vi "ttm_aecontrolnew_poller.vi"() -> ()   [LabVIEW 2011]
panel:
  out "On AE speed":bool=TRUE
  out "Axis Information Out":T1(array[cluster])
  out "Axis Selector Out":i32[](listbox)
  out "Channels Out":u16[](array[ring]) items=["Channel 1", "Channel 2", "Channel 3", "Channel 4"]
  out "Error Out":errorcluster
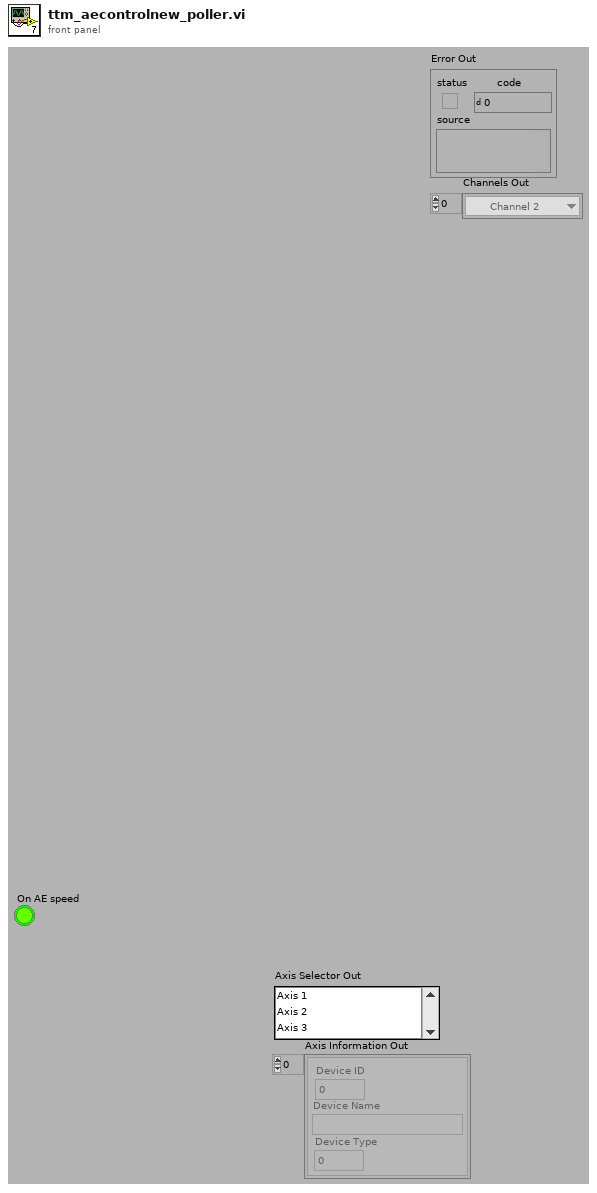
[diagram p1: front panel]
types:
  T1 = cluster{"Device ID":i32, "Device Name":string, "Device Type":i32}[]
  T2 = cluster{"Name":string, "Type":i32, "SI Full Scale":dbl, "Full Scale":dbl, "Units String":string, "Display Format":string, "Gauge Length":dbl}[][]
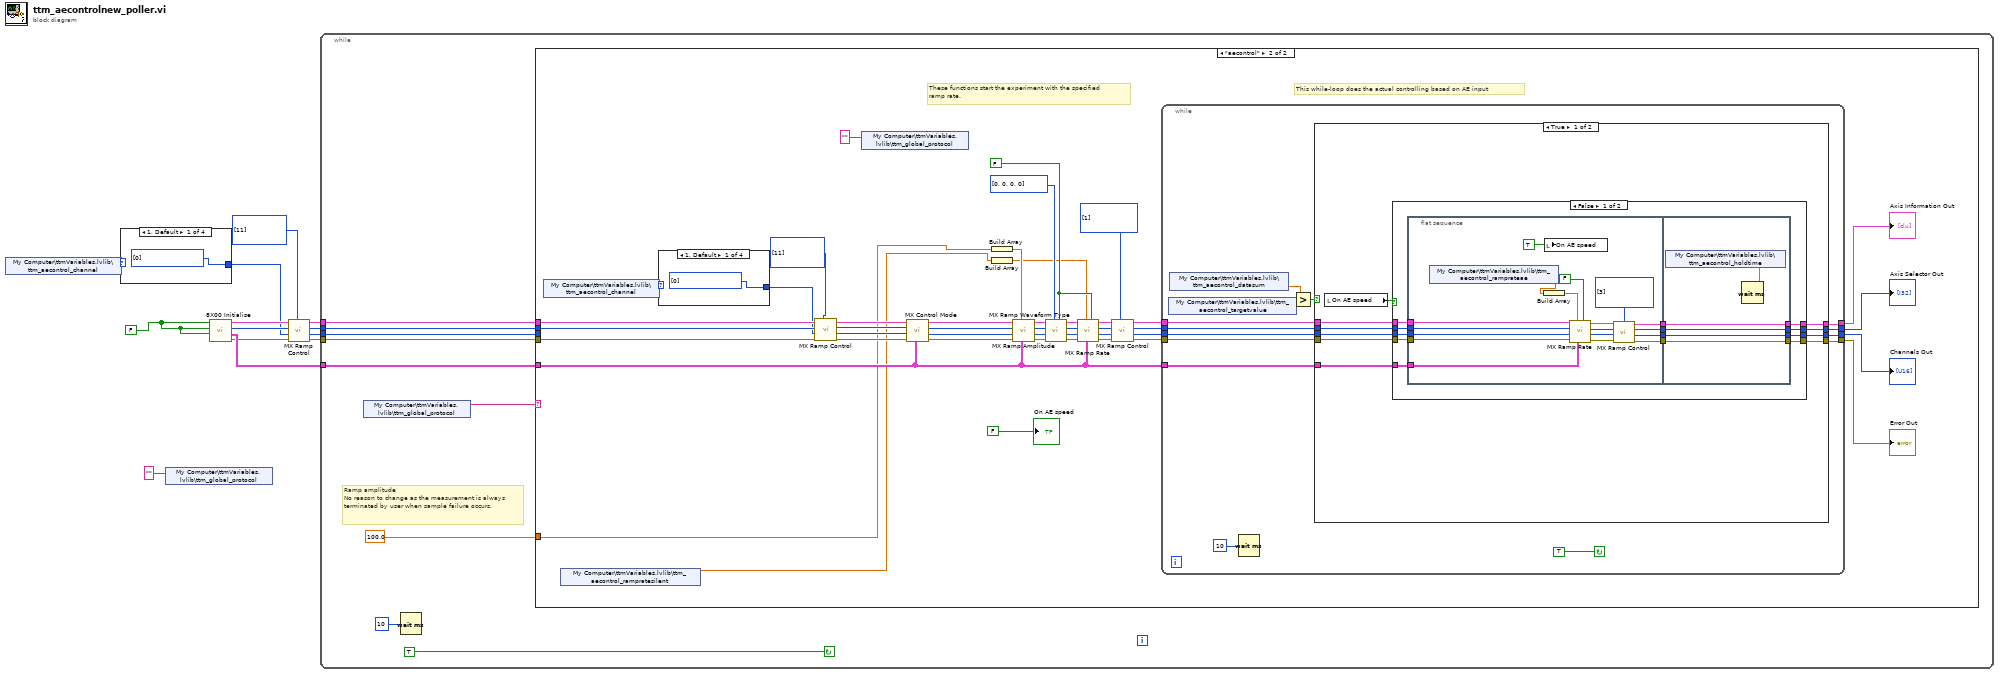
[diagram p0: block diagram]
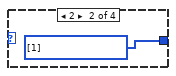
[diagram p2: hidden frame]
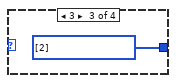
[diagram p3: hidden frame]
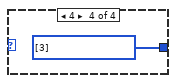
[diagram p4: hidden frame]
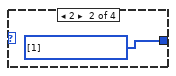
[diagram p6: hidden frame]
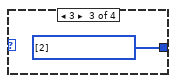
[diagram p7: hidden frame]
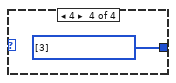
[diagram p8: hidden frame]
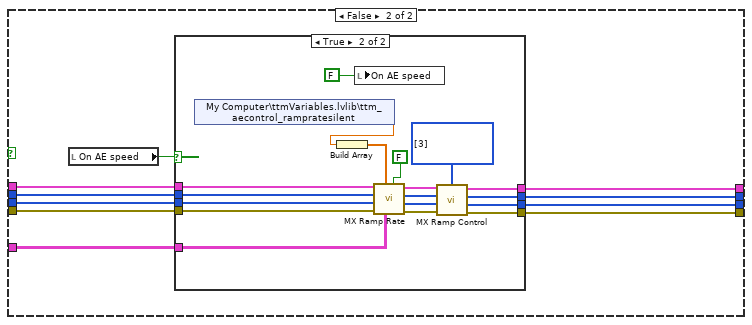
[diagram p10: hidden frame]
diagram:
  w7 = u16[] [11] items=["Stop", "Start or continue", "Hold", "Continue", "Return ramp to set level at fixed rate", "Reserved", "Reserved", "Start Random without demand hold", "Start Random with demand hold", "Prepare Random Start without demand hold", "Prepare Random Start with demand hold", "Unslave", "Reserved", "Reserved", "Start Sample Data Playback or Resume", "Prepare for Start of Sample Data", "Reserved", "Reserved", "Resume Playback", "Start an electromechanical frame return"] ("Ramp Control")
  w12 = FALSE ("Reset?")
  n1 = shared-variable "My Computer\\ttmVariables.lvlib\\ttm_aecontrol_channel"() -> (w9:i32)  [unwired: 1 in, 1 out]
  n2 = case shown="1, Default" w9 {
    tunnel: [w14 w15 w16 w17] -> w8
    frame 1, Default {
      w14 = u16[] [0] items=["Channel 1", "Channel 2", "Channel 3", "Channel 4"] ("Choose channel to apply\nthe setpoint")
    }
    frame 2 {
      w15 = u16[] [1] items=["Channel 1", "Channel 2", "Channel 3", "Channel 4"] ("Choose channel to apply\nthe setpoint")
    }
    frame 3 {
      w16 = u16[] [2] items=["Channel 1", "Channel 2", "Channel 3", "Channel 4"] ("Choose channel to apply\nthe setpoint")
    }
    frame 4 {
      w17 = u16[] [3] items=["Channel 1", "Channel 2", "Channel 3", "Channel 4"] ("Choose channel to apply\nthe setpoint")
    }
  }
  n3 = shared-variable "My Computer\\ttmVariables.lvlib\\ttm_global_protocol"("" ("protocol")) -> ()  [unwired: 1 in, 1 out]
  n4 = call "8X00 Initialise.vi"("Reset?"=w12, "Create DVM? (T)"=w12, "Create Console? (T)"=w12) -> ("error out"=w6:errorcluster, "Channel Data"=w13:T2, "Axis Selector"=w10:i32[], "Axis Information"=w11:T1)  [unwired: 1 in]
  n5 = call "MX Ramp Control.vi"("Ramp Control"=w7, "error in (no error)"=w6, "Channels In"=w8, "Axis Selector In"=w10, "Axis Information In"=w11) -> ("error out"=w2:errorcluster, "Channels Out"=w3:u16[], "Axis Selector Out"=w4:i32[], "Axis Information Out"=w5:T1)  [unwired: 2 in]
  n6 = while {
    tunnel: w13 -> [w25]
    tunnel: w5 -> [w22]
    tunnel: w4 -> [w21]
    tunnel: w3 -> [w20]
    tunnel: w2 -> [w19]
    stop <- TRUE continue-if-true
    # "Ramp amplitude\nNo reason to change as the measurement is always terminated by user when sample failure occurs."
    n7 = shared-variable "My Computer\\ttmVariables.lvlib\\ttm_global_protocol"() -> (w18:string)  [unwired: 1 in, 1 out]
    n8 = Wait (ms)(milliseconds to wait=u32 10) -> ()  [unwired: 1 out]
    n9 = case shown="\"aecontrol\"" w18 {
      tunnel: w25 -> [_ w41]
      tunnel: 100.0 ("rampAmplitude") -> [_ w28]
      tunnel: w22 -> [_ w37]
      tunnel: w21 -> [_ w36]
      tunnel: w20 -> [_ _]
      tunnel: w19 -> [_ w35]
      frame "False", Default {
      }
      frame "aecontrol" {
        w29 = u16[] [11] items=["Stop", "Start or continue", "Hold", "Continue", "Return ramp to set level at fixed rate", "Reserved", "Reserved", "Start Random without demand hold", "Start Random with demand hold", "Prepare Random Start without demand hold", "Prepare Random Start with demand hold", "Unslave", "Reserved", "Reserved", "Start Sample Data Playback or Resume", "Prepare for Start of Sample Data", "Reserved", "Reserved", "Resume Playback", "Start an electromechanical frame return"] ("Ramp Control")
        w50 = u16[] [1] items=["Stop", "Start or continue", "Hold", "Continue", "Return ramp to set level at fixed rate", "Reserved", "Reserved", "Start Random without demand hold", "Start Random with demand hold", "Prepare Random Start without demand hold", "Prepare Random Start with demand hold", "Unslave", "Reserved", "Reserved", "Start Sample Data Playback or Resume", "Prepare for Start of Sample Data", "Reserved", "Reserved", "Resume Playback", "Start an electromechanical frame return"] ("Ramp Control")
        w61 = FALSE ("Next?")
        w66 = u16[] [0, 0, 0, 0] items=["Ramp", "Dual Ramp", "Trapezium", "Absolute Ramp", "Hold Ramp", "Absolute Rate Ramp"] ("Waveform Types")
        # "This while-loop does the actual controlling based on AE input"
        # "These functions start the experiment with the specified\nramp rate."
        n10 = shared-variable "My Computer\\ttmVariables.lvlib\\ttm_aecontrol_channel"() -> (w31:i32)  [unwired: 1 in, 1 out]
        n11 = shared-variable "My Computer\\ttmVariables.lvlib\\ttm_aecontrol_rampratesilent"() -> (w27:dbl)  [unwired: 1 in, 1 out]
        n12 = case shown="1, Default" w31 {
          tunnel: [w71 w72 w73 w74] -> w30
          frame 1, Default {
            w71 = u16[] [0] items=["Channel 1", "Channel 2", "Channel 3", "Channel 4"] ("Choose channel to apply\nthe setpoint")
          }
          frame 2 {
            w72 = u16[] [1] items=["Channel 1", "Channel 2", "Channel 3", "Channel 4"] ("Choose channel to apply\nthe setpoint")
          }
          frame 3 {
            w73 = u16[] [2] items=["Channel 1", "Channel 2", "Channel 3", "Channel 4"] ("Choose channel to apply\nthe setpoint")
          }
          frame 4 {
            w74 = u16[] [3] items=["Channel 1", "Channel 2", "Channel 3", "Channel 4"] ("Choose channel to apply\nthe setpoint")
          }
        }
        n13 = call "MX Ramp Control.vi"("Ramp Control"=w29, "error in (no error)"=w35, "Channels In"=w30, "Axis Selector In"=w36, "Axis Information In"=w37) -> ("error out"=w34:errorcluster, "Channels Out"=w33:u16[], "Axis Selector Out"=w32:i32[], "Axis Information Out"=w38:T1)  [unwired: 2 in]
        n14 = shared-variable "My Computer\\ttmVariables.lvlib\\ttm_global_protocol"("" ("protocol")) -> ()  [unwired: 1 in, 1 out]
        n15 = call "MX Control Mode.vi"("Channel Data"=w41, "error in (no error)"=w34, "Control Modes"=w33, "Axis Selector"=w32, "Axis Information"=w38) -> ("error out"=w55:errorcluster, "Control Modes out"=w56:u16[], "Axis Selector out"=w57:i32[], "Axis Information out"=w58:T1)  [unwired: 1 in]
        n16 = Build Array(w28) -> (w60:dbl[])
        n17 = Build Array(w27) -> (w59:dbl[])
        n18 = call "MX Ramp Amplitude.vi"("Channel Data"=w41, "Ramp Amplitude"=w60, "error in (no error)"=w55, "Channels In"=w56, "Axis Selector In"=w57, "Axis Information In"=w58) -> ("error out"=w68:errorcluster, "Channels Out"=w69:u16[], "Axis Selector Out"=w70:i32[], "Axis Information Out"=w67:T1)  [unwired: 1 in]
        n19 = call "MX Ramp Waveform Type.vi"("Next?"=w61, "Waveform Types"=w66, "error in (no error)"=w68, "Channels In"=w69, "Axis Selector In"=w70, "Axis Information In"=w67) -> ("error out"=w62:errorcluster, "Channels Out"=w63:u16[], "Axis Selector Out"=w64:i32[], "Axis Information Out"=w65:T1)  [unwired: 1 in]
        n20 = call "MX Ramp Rate.vi"("Next?"=w61, "Channel Data"=w41, "Ramp Rate"=w59, "error in (no error)"=w62, "Channels In"=w63, "Axis Selector In"=w64, "Axis Information In"=w65) -> ("error out"=w51:errorcluster, "Channels Out"=w52:u16[], "Axis Selector Out"=w53:i32[], "Axis Information Out"=w54:T1)
        n21 = call "MX Ramp Control.vi"("Ramp Control"=w50, "error in (no error)"=w51, "Channels In"=w52, "Axis Selector In"=w53, "Axis Information In"=w54) -> ("error out"=w46:errorcluster, "Channels Out"=w47:u16[], "Axis Selector Out"=w48:i32[], "Axis Information Out"=w49:T1)  [unwired: 2 in]
        n22 = while {
          tunnel: w49 -> [w87]
          tunnel: w48 -> [w86]
          tunnel: w47 -> [w85]
          tunnel: w46 -> [w84]
          tunnel: [w83] -> w45
          tunnel: [w82] -> w44
          tunnel: [w81] -> w43
          tunnel: [w80] -> w42
          tunnel: w41 -> [w78]
          stop <- TRUE continue-if-true
          n23 = shared-variable "My Computer\\ttmVariables.lvlib\\ttm_aecontrol_targetvalue"() -> (w76:dbl)  [unwired: 1 in, 1 out]
          n24 = shared-variable "My Computer\\ttmVariables.lvlib\\ttm_aecontrol_datasum"() -> (w77:dbl)  [unwired: 1 in, 1 out]
          n25 = Wait (ms)(milliseconds to wait=u32 10) -> ()  [unwired: 1 out]
          n26 = Greater?(x=w77, y=w76) -> (0:w75:bool)
          n27 = case shown="True" w75 {
            tunnel: w87 -> [w98 w148]
            tunnel: w86 -> [w97 w147]
            tunnel: w85 -> [w96 w146]
            tunnel: w84 -> [w95 w145]
            tunnel: [w94 w144] -> w83
            tunnel: [w93 w143] -> w82
            tunnel: [w92 w142] -> w81
            tunnel: [w91 w141] -> w80
            tunnel: w78 -> [w90 w140]
            frame True {
              n28 = local read "On AE speed"() -> (w89:bool)
              n29 = case shown="False" w89 {
                tunnel: w98 -> [w111 w138]
                tunnel: w97 -> [w110 w137]
                tunnel: w96 -> [w109 w136]
                tunnel: w95 -> [w108 w135]
                tunnel: [w107 w138] -> w94
                tunnel: [w106 w137] -> w93
                tunnel: [w105 w136] -> w92
                tunnel: [w104 w135] -> w91
                tunnel: w90 -> [w103 _]
                frame False {
                  n30 = flat-sequence {
                    tunnel: w111 -> [w129]
                    tunnel: w110 -> [w128]
                    tunnel: w109 -> [w127]
                    tunnel: w108 -> [w126]
                    tunnel: w103 -> [w114]
                    tunnel: [w119] -> w102
                    tunnel: [w118] -> w101
                    tunnel: [w117] -> w100
                    tunnel: [w116] -> w99
                    tunnel: [w131] -> w104
                    tunnel: [w132] -> w105
                    tunnel: [w133] -> w106
                    tunnel: [w134] -> w107
                    tunnel: w102 -> [w134]
                    tunnel: w101 -> [w133]
                    tunnel: w100 -> [w132]
                    tunnel: w99 -> [w131]
                    frame #0 {
                      w115 = u16[] [3] items=["Stop", "Start or continue", "Hold", "Continue", "Return ramp to set level at fixed rate", "Reserved", "Reserved", "Start Random without demand hold", "Start Random with demand hold", "Prepare Random Start without demand hold", "Prepare Random Start with demand hold", "Unslave", "Reserved", "Reserved", "Start Sample Data Playback or Resume", "Prepare for Start of Sample Data", "Reserved", "Reserved", "Resume Playback", "Start an electromechanical frame return"] ("Ramp Control")
                      n31 = shared-variable "My Computer\\ttmVariables.lvlib\\ttm_aecontrol_ramprateae"() -> (w112:dbl)  [unwired: 1 in, 1 out]
                      n32 = Build Array(w112) -> (w124:dbl[])
                      n33 = local write "On AE speed"(TRUE ("On AE speed")) -> ()
                      n34 = call "MX Ramp Rate.vi"("Next?"=FALSE, "Channel Data"=w114, "Ramp Rate"=w124, "error in (no error)"=w126, "Channels In"=w127, "Axis Selector In"=w128, "Axis Information In"=w129) -> ("error out"=w120:errorcluster, "Channels Out"=w121:u16[], "Axis Selector Out"=w122:i32[], "Axis Information Out"=w123:T1)
                      n35 = call "MX Ramp Control.vi"("Ramp Control"=w115, "error in (no error)"=w120, "Channels In"=w121, "Axis Selector In"=w122, "Axis Information In"=w123) -> ("error out"=w116:errorcluster, "Channels Out"=w117:u16[], "Axis Selector Out"=w118:i32[], "Axis Information Out"=w119:T1)  [unwired: 2 in]
                    }
                    frame #1 {
                      n36 = shared-variable "My Computer\\ttmVariables.lvlib\\ttm_aecontrol_holdtime"() -> (w130:dbl)  [unwired: 1 in, 1 out]
                      n37 = Wait (ms)(milliseconds to wait=w130) -> ()  [unwired: 1 out]
                    }
                  }
                }
                frame True {
                }
              }
            }
            frame False {
              n38 = local read "On AE speed"() -> (w139:bool)
              n39 = case shown="True" w139 {
                tunnel: w148 -> [w152 w170]
                tunnel: w147 -> [w151 w169]
                tunnel: w146 -> [w150 w168]
                tunnel: w145 -> [w149 w167]
                tunnel: [w152 w160] -> w144
                tunnel: [w151 w159] -> w143
                tunnel: [w150 w158] -> w142
                tunnel: [w149 w157] -> w141
                tunnel: w140 -> [_ w155]
                frame False {
                }
                frame True {
                  w156 = u16[] [3] items=["Stop", "Start or continue", "Hold", "Continue", "Return ramp to set level at fixed rate", "Reserved", "Reserved", "Start Random without demand hold", "Start Random with demand hold", "Prepare Random Start without demand hold", "Prepare Random Start with demand hold", "Unslave", "Reserved", "Reserved", "Start Sample Data Playback or Resume", "Prepare for Start of Sample Data", "Reserved", "Reserved", "Resume Playback", "Start an electromechanical frame return"] ("Ramp Control")
                  n40 = shared-variable "My Computer\\ttmVariables.lvlib\\ttm_aecontrol_rampratesilent"() -> (w153:dbl)  [unwired: 1 in, 1 out]
                  n41 = Build Array(w153) -> (w165:dbl[])
                  n42 = local write "On AE speed"(FALSE ("On AE speed")) -> ()
                  n43 = call "MX Ramp Rate.vi"("Next?"=FALSE, "Channel Data"=w155, "Ramp Rate"=w165, "error in (no error)"=w167, "Channels In"=w168, "Axis Selector In"=w169, "Axis Information In"=w170) -> ("error out"=w161:errorcluster, "Channels Out"=w162:u16[], "Axis Selector Out"=w163:i32[], "Axis Information Out"=w164:T1)
                  n44 = call "MX Ramp Control.vi"("Ramp Control"=w156, "error in (no error)"=w161, "Channels In"=w162, "Axis Selector In"=w163, "Axis Information In"=w164) -> ("error out"=w157:errorcluster, "Channels Out"=w158:u16[], "Axis Selector Out"=w159:i32[], "Axis Information Out"=w160:T1)  [unwired: 2 in]
                }
              }
            }
          }
        }
        "Error Out" <- w42
        "Channels Out" <- w43
        "Axis Selector Out" <- w44
        "Axis Information Out" <- w45
        "On AE speed" <- FALSE ("On AE speed")
      }
    }
  }
